vi "Wire Event Data Out.vi"(8 "error in (no error)":errorcluster, 9 "Event Data Names":string[](array[string]), 10 "Event Data":refnum<vi>[](array[refnum]), 11 "Diagram in":refnum<vi>) -> (0 "error out":errorcluster, 3 "Diagram out":refnum<vi>)   [LabVIEW 2015, in "Scripting.lvlib"]
uses:
  Scripting.lvlib
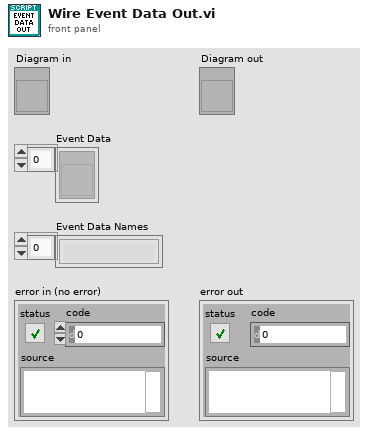
[diagram p1: front panel]
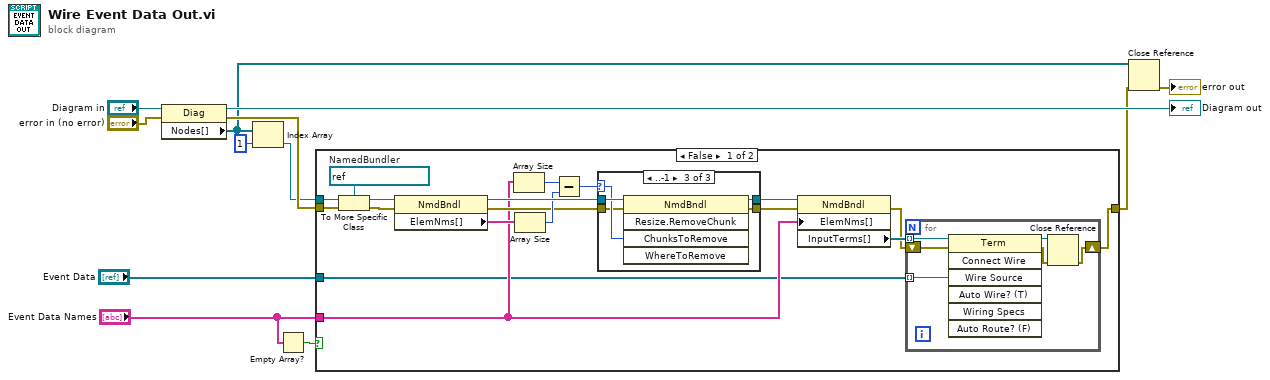
[diagram p0: block diagram]
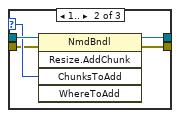
[diagram p3: hidden frame]
diagram:
  n1 = property class="Diag"(reference="Diagram in", error in="error in (no error)") -> (reference out=→"Diagram out":refnum<vi>, error out=w12:errorcluster, "Nodes[]"=w3:refnum<vi>[])
  n2 = Index Array(array=w3, index=1) -> (element=w8:refnum<vi>)
  n3 = Empty Array?(array="Event Data Names") -> (empty?=w10:bool)
  n4 = case shown="False" w10 {
    tunnel: w8 -> [w30 _]
    tunnel: w12 -> [w29 w49]
    tunnel: "Event Data Names" -> [w17 _]
    tunnel: [w13 w49] -> w2
    tunnel: "Event Data" -> [w15 _]
    frame False {
      w28 = refnum<vi> refnum  # NamedBundler
      n5 = To More Specific Class(target class=w28, reference=w30, error in=w29) -> (specific class reference=w22:refnum<vi>, error out=w19:errorcluster)
      n6 = property class="NmdBndl"(reference=w22, error in=w19) -> (reference out=w27:refnum<vi>, error out=w18:errorcluster, "ElemNms[]"=w26:string[])
      n7 = Array Size(array=w17) -> (size(s)=w24:i32)
      n8 = Array Size(array=w26) -> (size(s)=w25:i32)
      n9 = Subtract(x=w24, y=w25) -> (x-y=w23:i32)
      n10 = case shown="..-1" w23 {
        selector: w23 -> [_ w42 w47]
        tunnel: w27 -> [w38 w43 w48]
        tunnel: [w38 w41 w46] -> w21
        tunnel: w18 -> [w37 w40 w44]
        tunnel: [w37 w39 w45] -> w20
        frame 0 {
        }
        frame 1.. {
          n11 = invoke class="NmdBndl" method="Resize.AddChunk"(reference=w43, error in=w40, "ChunksToAdd"=w42) -> (reference out=w41:refnum<vi>, error out=w39:errorcluster)  [unwired: 2 in, 3 out]
        }
        frame ..-1 {
          n12 = invoke class="NmdBndl" method="Resize.RemoveChunk"(reference=w48, error in=w44, "ChunksToRemove"=w47) -> (reference out=w46:refnum<vi>, error out=w45:errorcluster)  [unwired: 2 in, 3 out]
        }
      }
      n13 = property class="NmdBndl"(reference=w21, error in=w20, "ElemNms[]"=w17) -> (error out=w14:errorcluster, "InputTerms[]"=w16:refnum<vi>[])  [unwired: 1 out]
      n14 = for {
        tunnel: w16 -> [w36] mode=indexing
        tunnel: w15 -> [w35] mode=indexing
        shift-right: [w32] -> w13
        shift-left: w14 -> [w34]
        n15 = invoke class="Term" method="Connect Wire"(reference=w36, error in=w34, "Wire Source"=w35) -> (reference out=w31:refnum<vi>, error out=w33:errorcluster)  [unwired: 4 in, 5 out]
        n16 = Close Reference(reference=w31, error in (no error)=w33) -> (error out=w32:errorcluster)
      }
    }
    frame True {
    }
  }
  n17 = Close Reference(reference=w3, error in (no error)=w2) -> (error out=→"error out":errorcluster)
